vi "FFT.vi"() -> ()   [LabVIEW 2020]
uses:
  <vilib>/rvi/Analysis/measure/FFT/simModelSupport/niFPGA FFT Outside SCTL Sim Properties.ctl
  <vilib>/rvi/Analysis/measure/FFT/simModelSupport/niFPGA FFT Sim Types.ctl
  <vilib>/rvi/Analysis/measure/FFT/simModelSupport/niFpgaFFTSimArithmeticProperties.ctl
  <vilib>/rvi/Analysis/measure/FFT/simModelSupport/niFpgaFFTSimDfxp.ctl
  <vilib>/fxp/LVFixedPointQuantizationPolicyTypeDef.ctl
  <vilib>/rvi/DataTransferAndStorage/Container/Common/niFpgaContainerGetUniqueNameForEmu.vi
  <vilib>/rvi/DataTransferAndStorage/Container/Common/niFpgaContainerSetEmuInfo.vi
  <vilib>/rvi/eio/common/nirviEmuReportErrorAndStop.vi
  <vilib>/rvi/interface/RandomDataEmulation/niFpgaRandomDataHandleErrors.vi
  <vilib>/rvi/DataTransferAndStorage/Container/Common/niFpgaContainerExecOnDevCompGetState.vi
  <vilib>/rvi/Emulation/niFpgaEmulationIsFPGAContextNoSignature.vi
  <vilib>/rvi/Emulation/niFpgaSctlEmulationGetInTimedLoop.vi
  <vilib>/rvi/errors/niFpgaSetErrorForExecOnDevCompSimple.vi
  <vilib>/rvi/FIFO/Fifo_Resource/nirvififoEmulationSetSize.vi
  <vilib>/rvi/FIFO/Fifo_Resource/nirviFifoEmulationQueueMgr.vi
  <instcachedir>/0/nirviFifoEmulationQueueMgr_E5CAEC123FF24DC58D834DCA3CDAA9B5.lvgen/nirviFifoEmulationQueueMgr_E5CAEC123FF24DC58D834DCA3CDAA9B5_008.vi
  <vilib>/rvi/FIFO/Fifo_Resource/nirvififoEmulationDetermineInputValidOut.vi
  <vilib>/rvi/FIFO/Fifo_Resource/nirvififoEmulationCreateLock.vi
  <vilib>/rvi/Emulation/niFpgaProcessEmulError.vi
  <vilib>/rvi/FIFO/Fifo_Resource/nirvififoEmulationObtainLock.vi
  <vilib>/rvi/FIFO/Fifo_Resource/nirvififoEmulationReleaseLock.vi
  <vilib>/rvi/occurrence/nirviWaitOnOccurrenceBase.vi
  <vilib>/rvi/errors/nirviReportUnexpectedCaseInternalError.vi
  <vilib>/rvi/errors/nirviReportUnexpectedCaseInternalError (U32).vi
  <vilib>/Utility/error.llb/Clear Errors.vi
  <vilib>/rvi/Emulation/niFpgaGetClockAttributes.vi
  <vilib>/rvi/Emulation/niFpgaEmulationReportErrorSimple.vi
  <vilib>/rvi/Analysis/measure/FFT/simModelSupport/niFpgaFFTSimModelOutsideSCTLCore.vi
  <vilib>/rvi/Emulation/niFpgaCriticalErrorInLSC.vi
  <vilib>/rvi/LocalResourceManager/LocalResourceManager.xnode
  <vilib>/rvi/DataTransferAndStorage/Container/XNode/niFpgaContainer.xnode
  <vilib>/rvi/interface/RandomDataEmulation/nirviRandomDataFpgaReadWriteTemplate.vi
  <vilib>/rvi/FIFO/Fifo_Resource/niFpgaFifoEmulationRefIn.vi
  <vilib>/rvi/Analysis/measure/FFT/XNode/niFpgaFFT.xnode
panel:
  out "Numeric":i32
  out "appended array":fxp<+/-,24,7>[](array[numeric])
  out "x-y (microsecond)":u32
  out "data index":u16
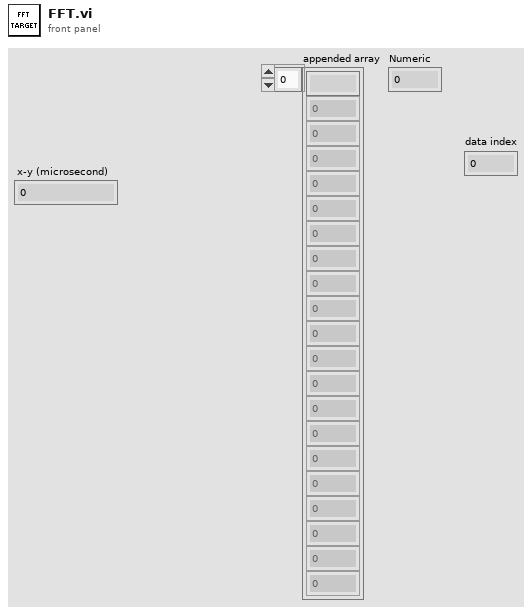
[diagram p1: front panel]
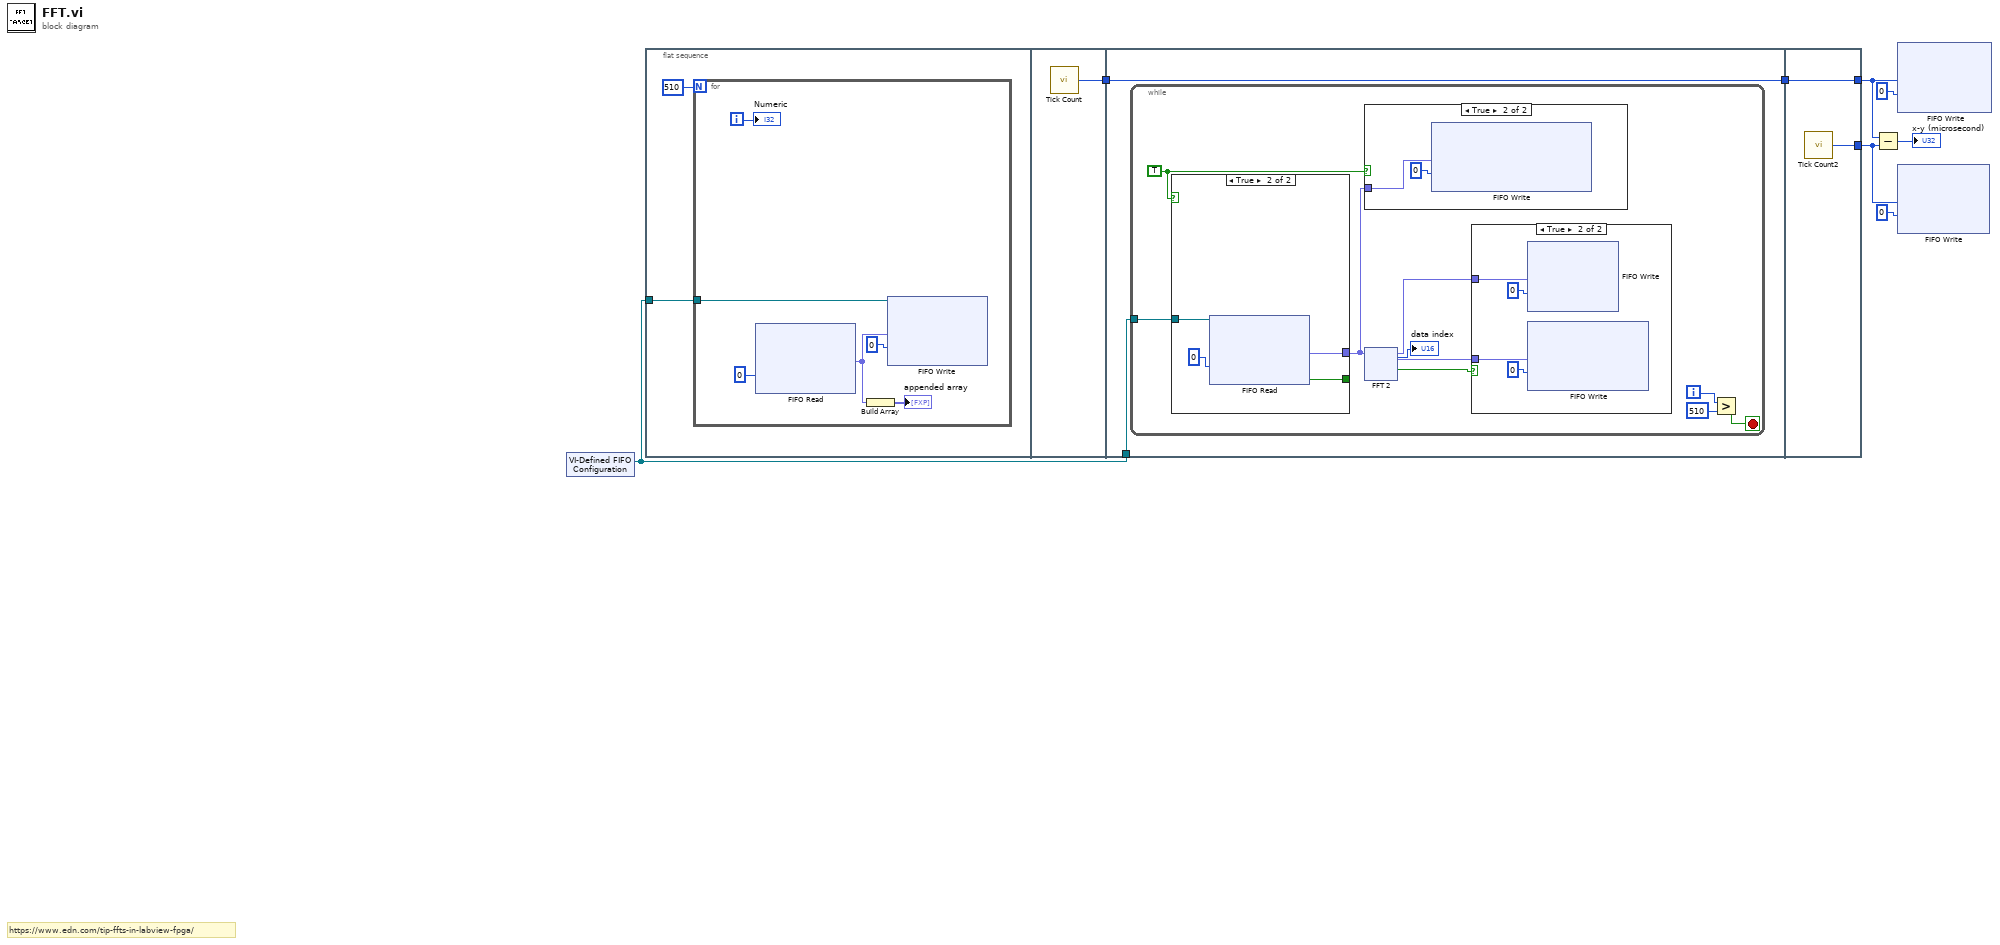
[diagram p0: block diagram]
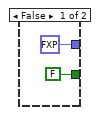
[diagram p3: hidden frame]
diagram:
  # "https://www.edn.com/tip-ffts-in-labview-fpga/"
  n1 = xnode "VI-Defined FIFO Configuration"() -> ("FIFO Out"=w1:refnum<k21>)
  n2 = flat-sequence {
    tunnel: w1 -> [w10]
    tunnel: [w17] -> w8
    tunnel: [w19] -> w7
    tunnel: w8 -> [w19]
    tunnel: w1 -> [w18]
    tunnel: [w63] -> w5
    tunnel: w7 -> [w63]
    tunnel: [w62] -> w4
    frame #0 {
      n3 = for {
        N: 510 -> [_]
        tunnel: w10 -> [w15]
        i -> [w11]
        n4 = xnode ("FIFO Read")("Timeout"=0) -> ("Element"=w13:fxp<+/-,24,7>)  [unwired: 1 in, 2 out]
        n5 = Build Array(w13) -> (→"appended array":fxp<+/-,24,7>[])
        n6 = xnode ("FIFO Write")("Element"=w13, "Timeout"=0, "FIFO In"=w15) -> ()  [unwired: 2 out]
        "Numeric" <- w11
      }
    }
    frame #1 {
      n7 = call "Tick Count"() -> ("Tick Count(uSec)"=w17:u32)
    }
    frame #2 {
      n8 = while {
        tunnel: w18 -> [w20]
        i -> [w26]
        stop <- w27 stop-if-true
        w21 = TRUE ("ready for input")
        n9 = case shown="True" w21 {
          tunnel: [fxp<+/-,24,7> 0.0 ("Element") w35] -> w22
          tunnel: [FALSE ("Timed Out?") w34] -> _
          tunnel: w20 -> [_ w37]
          frame False {
          }
          frame True {
            n10 = xnode ("FIFO Read")("Timeout"=0, "FIFO In"=w37) -> ("Element"=w35:fxp<+/-,24,7>, "Timed Out?"=w34:bool)  [unwired: 1 out]
          }
        }
        n11 = case shown="True" w21 {
          tunnel: w22 -> [_ w31]
          frame False {
          }
          frame True {
            n12 = xnode ("FIFO Write")("Element"=w31, "Timeout"=0) -> ()  [unwired: 1 in, 2 out]
          }
        }
        n13 = xnode ("FFT 2")("real data in"=w22) -> ("data index"=→"data index":u16, "real data out"=w25:fxp<+/-,32,15>, "imaginary data out"=w24:fxp<+/-,32,15>, "output valid"=w28:bool)  [unwired: 2 in]
        n14 = case shown="True" w28 {
          tunnel: w24 -> [_ w38]
          tunnel: w25 -> [_ w39]
          frame False {
          }
          frame True {
            n15 = xnode ("FIFO Write")("Element"=w39, "Timeout"=0) -> ()  [unwired: 1 in, 2 out]
            n16 = xnode ("FIFO Write")("Element"=w38, "Timeout"=0) -> ()  [unwired: 1 in, 2 out]
          }
        }
        n17 = Greater?(x=w26, y=510 ("Timeout")) -> (0:w27:bool)
      }
    }
    frame #3 {
      n18 = call "Tick Count2"() -> ("Tick Count(uSec)"=w62:u32)
    }
  }
  n19 = Subtract(x=w5, y=w4) -> (x-y=→"x-y (microsecond)":u32)
  n20 = xnode ("FIFO Write")("Element"=w5, "Timeout"=0) -> ()  [unwired: 1 in, 2 out]
  n21 = xnode ("FIFO Write")("Element"=w4, "Timeout"=0) -> ()  [unwired: 1 in, 2 out]
